vi "Data_Partitioning log.vi"() -> ()   [LabVIEW 2020]
uses:
  Global Variables/Trial_Flag.vi
  Global Variables/Global Send To ANN.vi
  Global Variables/Trainning Done.vi
  Global Variables/rating_done.vi
  Global Variables/Global User_Answer.vi
panel:
  out "Array of Single":sgl[][](array[numeric])
  out "Sended frame":dbl[](array[numeric])
  out "sorted 2D array":dbl[][](array[numeric])
  out "Open File":errorcluster
  out "Pre-Partition":dbl[][](array[numeric])
  in  "stop":bool
  # "Correct"
  # "Trial n"
  # "Window n"
  # "Timestamp"
  # "Left pupil"
  # "Right pupil"
  # "Label"
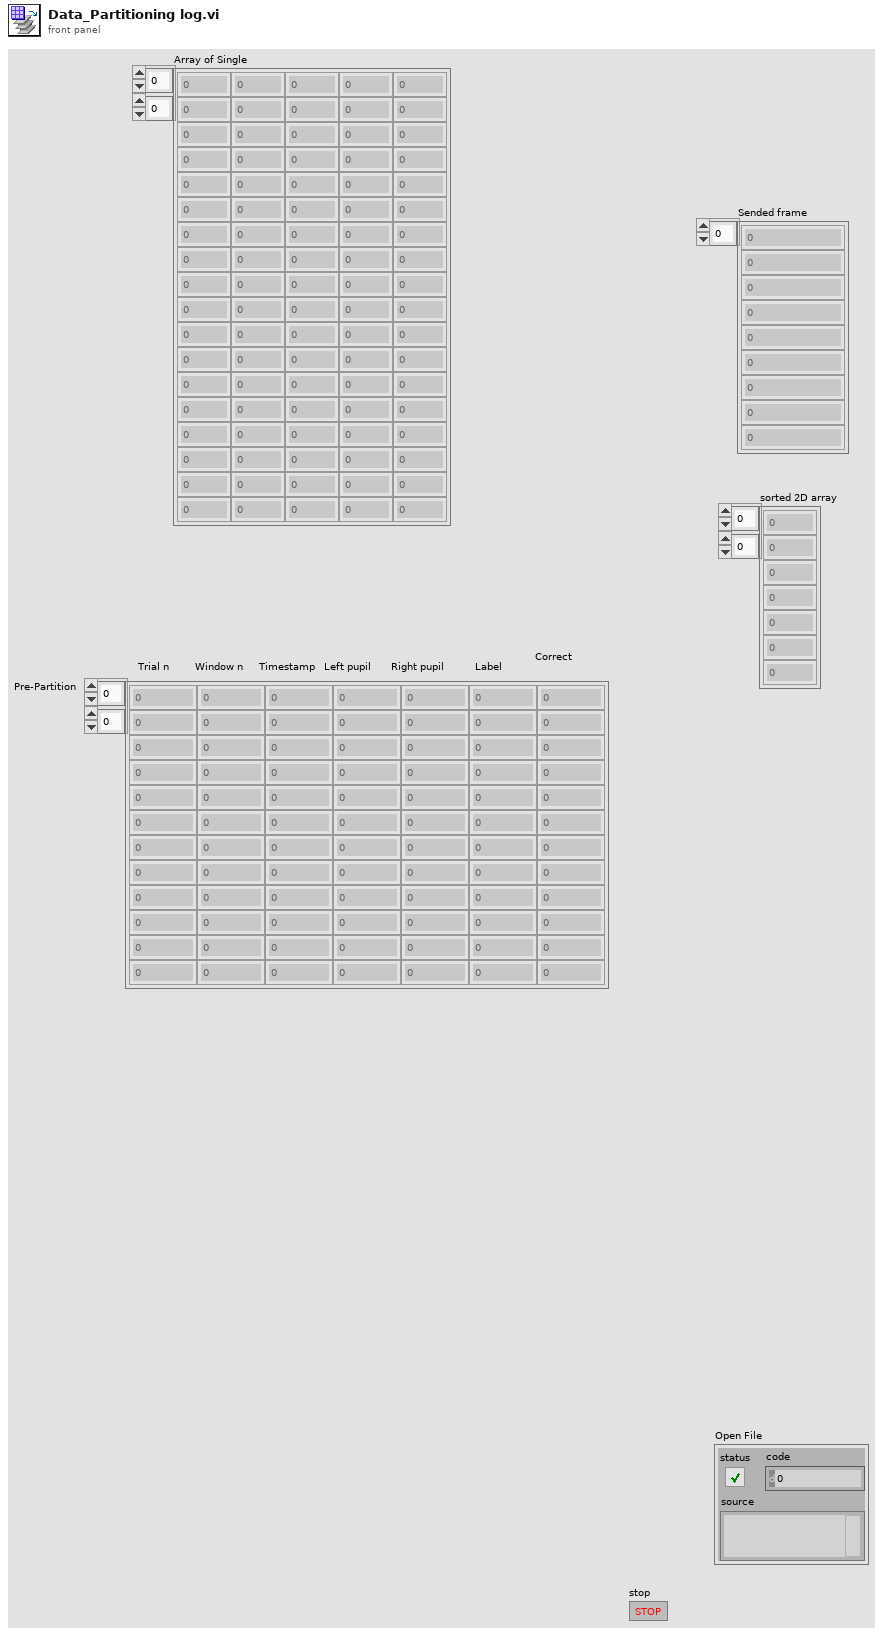
[diagram p1: front panel]
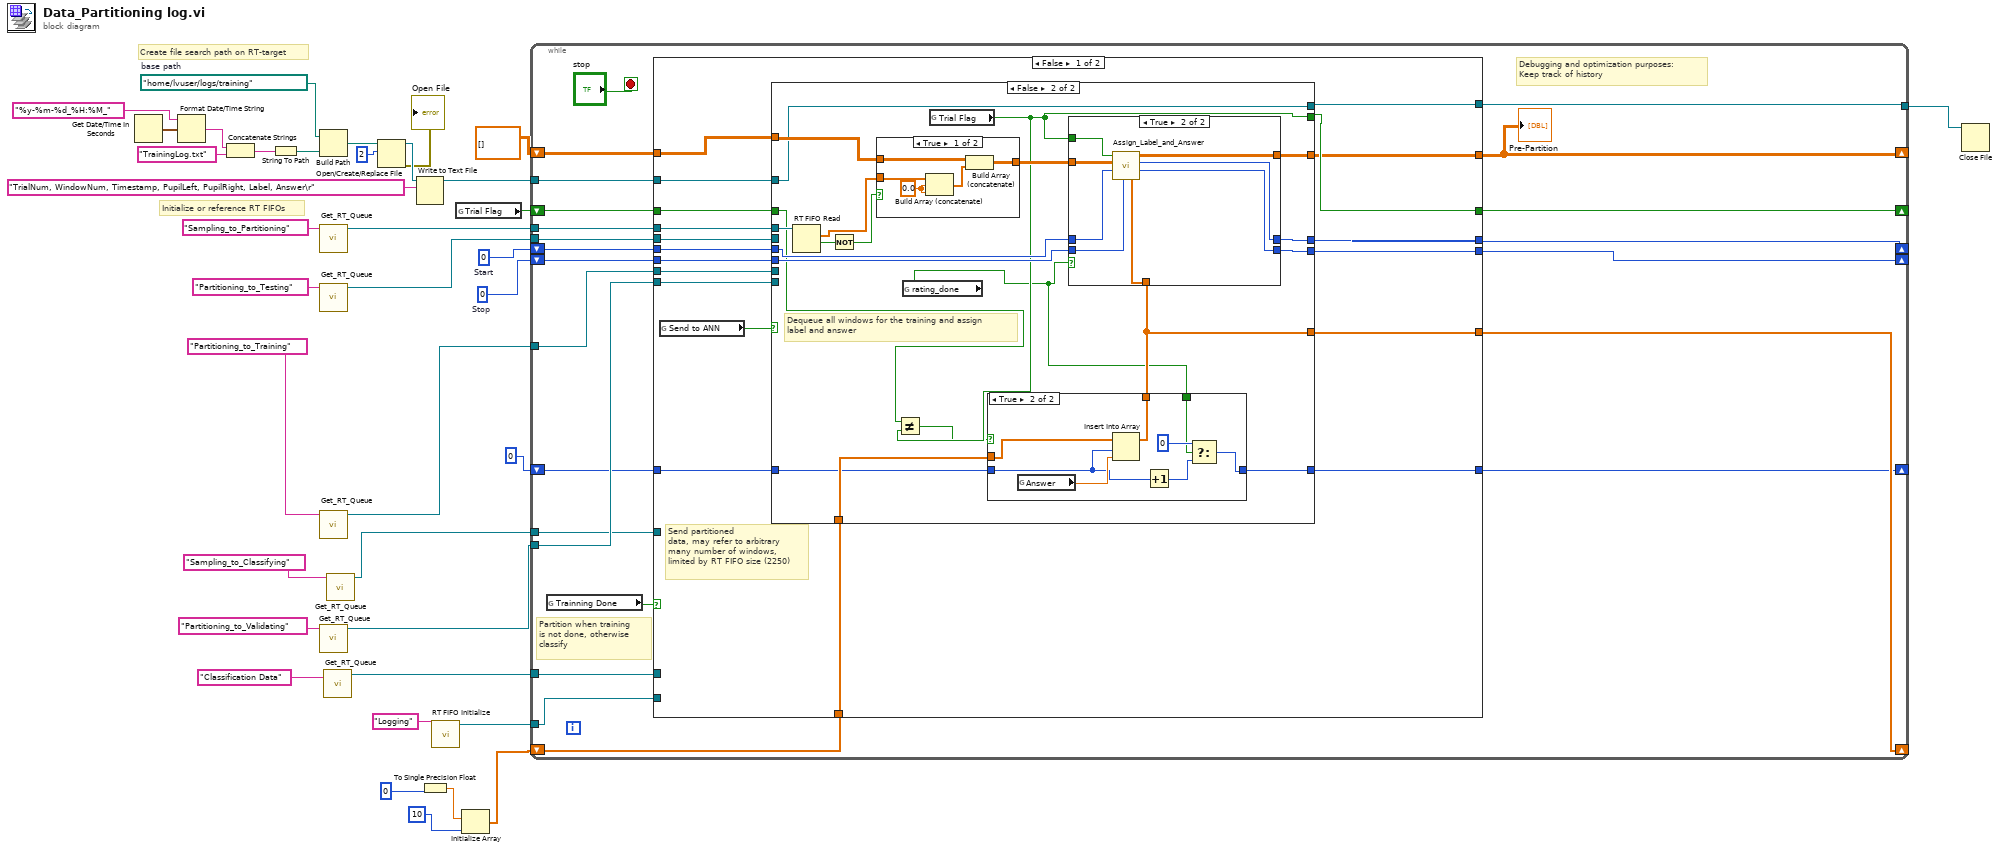
[diagram p0: block diagram]
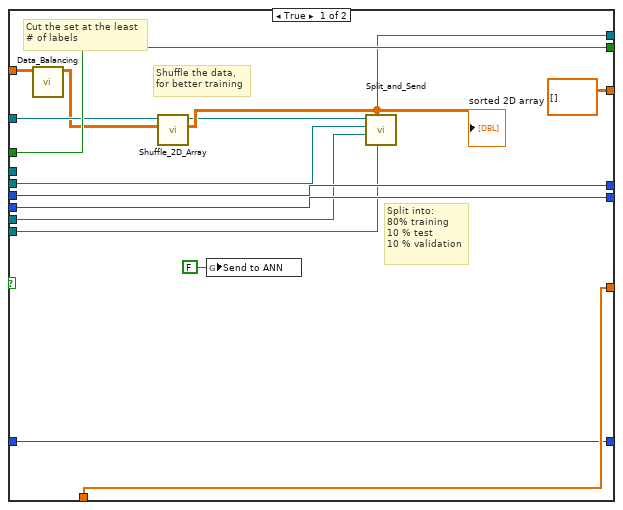
[diagram p2: hidden frame]
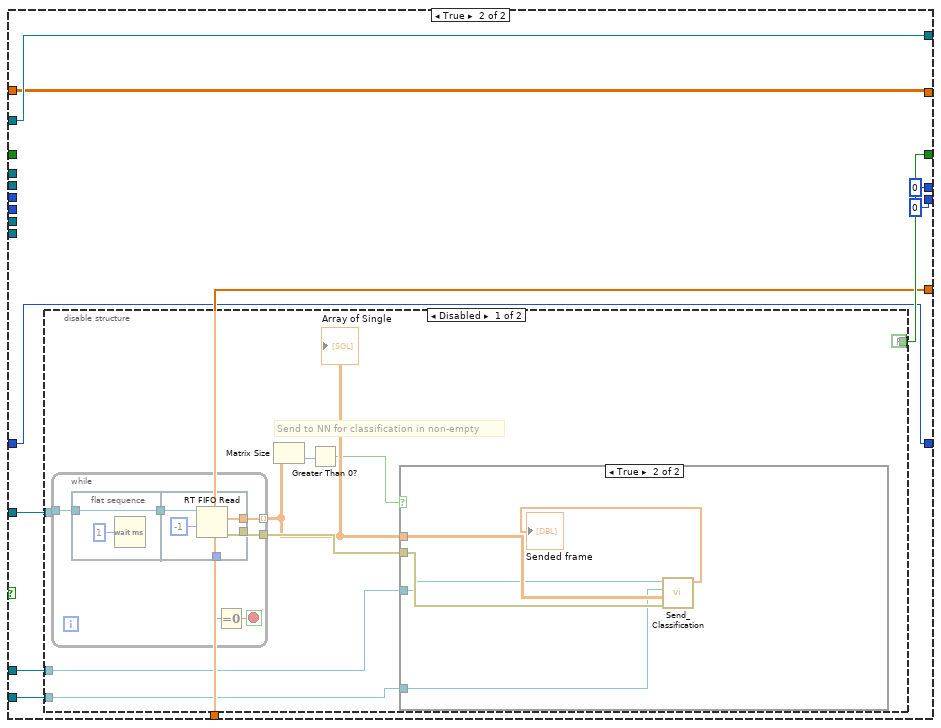
[diagram p6: hidden frame]
diagram:
  w32 = path "/home/lvuser/logs/training"  # base path
  w37 = 0  # Start
  w36 = 0  # Stop
  # "Initialize or reference RT FIFOs"
  # "Create file search path on RT-target"
  n1 = Get Date/Time In Seconds() -> (seconds since 1Jan1904=w25:timestamp)
  n2 = Format Date/Time String(time format string (%c)="%y-%m-%d_%H:%M_", seconds (now)=w25) -> (date/time string=w24:string)  [unwired: 1 in]
  n3 = Concatenate Strings(w24, "TrainingLog.txt") -> (w29:string)
  n4 = String To Path(string=w29) -> (path=w30:path)
  n5 = Build Path(base path=w32, name or relative path=w30) -> (appended path=w33:path)
  n6 = call "Get_RT_Queue.vi"("String"="Sampling_to_Partitioning") -> ("rt fifo single"=w13:refnum<k33>)  [unwired: 8 in, 2 out]
  n7 = call "Get_RT_Queue.vi"("String"="Partitioning_to_Testing") -> ("rt fifo single"=w15:refnum<k33>)  [unwired: 8 in, 2 out]
  n8 = call "Get_RT_Queue.vi"("String"="Partitioning_to_Training") -> ("rt fifo single"=w18:refnum<k33>)  [unwired: 8 in, 2 out]
  n9 = call "Get_RT_Queue.vi"("String"="Partitioning_to_Validating") -> ("rt fifo single"=w19:refnum<k33>)  [unwired: 8 in, 2 out]
  n10 = call "Get_RT_Queue.vi"("String"="Classification Data") -> ("rt fifo single"=w8:refnum<k33>)  [unwired: 8 in, 2 out]
  n11 = call "Get_RT_Queue.vi"("String"="Sampling_to_Classifying") -> ("rt fifo single"=w9:refnum<k33>)  [unwired: 8 in, 2 out]
  n12 = Open/Create/Replace File(file path (use dialog)=w33, operation (0:open)=2) -> (refnum out=w34:refnum<file>, error out=→"Open File":errorcluster)  [unwired: 4 in, 1 out]
  n13 = Write to Text File(file (use dialog)=w34, text="TrialNum, WindowNum, Timestamp, PupilLeft, PupilRight, Label, Answer\r") -> (refnum out=w27:refnum<file>)  [unwired: 2 in, 2 out]
  n14 = To Single Precision Float(number=0) -> (single precision float=w3:sgl)
  n15 = call "RT FIFO Initialize.vi"("name (unnamed)"="Logging") -> ("rt fifo"=w6:refnum<k33>)  [unwired: 9 in, 1 out]
  n16 = global read "Trial_Flag.vi" "Trial Flag"() -> (w35:bool)
  n17 = Initialize Array(w3, 10) -> (w2:sgl[])
  n18 = while {
    shift-right: [w47] -> _
    shift-left: sgl[][] [] -> [w60]
    shift-right: [w57] -> _
    shift-left: w37 -> [w55]
    shift-right: [w58] -> _
    shift-left: w36 -> [w46]
    shift-right: [w54] -> _
    shift-left: w35 -> [w56]
    tunnel: w13 -> [w53]
    tunnel: w18 -> [w52]
    tunnel: w15 -> [w51]
    tunnel: w19 -> [w50]
    tunnel: w27 -> [w49]
    tunnel: [w48] -> w22
    tunnel: w8 -> [w44]
    tunnel: w9 -> [w43]
    tunnel: w6 -> [w42]
    shift-right: [w39] -> _
    shift-left: w2 -> [w41]
    shift-right: [w38] -> _
    shift-left: 0 -> [w40]
    stop <- "stop" stop-if-true
    # "Debugging and optimization purposes: \nKeep track of history"
    # "Partition when training \nis not done, otherwise \nclassify"
    n19 = global read "Trainning Done.vi" "Trainning Done"() -> (w45:bool)
    n20 = case shown="False" w45 {
      tunnel: w60 -> [w79 w148]
      tunnel: [w78 0 ("Start out")] -> w58
      tunnel: [w77 0 ("Stop out")] -> w57
      tunnel: w56 -> [w76 _]
      tunnel: w55 -> [w75 _]
      tunnel: [w74 w150] -> w54
      tunnel: w53 -> [w73 _]
      tunnel: w52 -> [w72 _]
      tunnel: w51 -> [w71 _]
      tunnel: w50 -> [w70 _]
      tunnel: w49 -> [w69 w149]
      tunnel: [w68 w149] -> w48
      tunnel: [w67 w148] -> w47
      tunnel: w46 -> [w66 _]
      tunnel: w44 -> [_ w146]
      tunnel: w43 -> [_ w147]
      tunnel: w42 -> [_ w145]
      tunnel: w41 -> [w64 w144]
      tunnel: w40 -> [w63 w143]
      tunnel: [w62 w144] -> w39
      tunnel: [w61 w143] -> w38
      frame False {
        # "Send partitioned \ndata, may refer to arbitrary \nmany number of windows, \nlimited by RT FIFO size (2250)"
        n21 = global read "Global Send To ANN.vi" "Send to ANN"() -> (w65:bool)
        n22 = case shown="False" w65 {
          tunnel: w79 -> [w85 w115]
          tunnel: [w94 w113] -> w78
          tunnel: [sgl[][] [] ("Array out") w112] -> w67
          tunnel: [w93 w111] -> w77
          tunnel: w76 -> [w95 w103]
          tunnel: w75 -> [w93 w110]
          tunnel: w66 -> [w94 w109]
          tunnel: [w95 w102] -> w74
          tunnel: w73 -> [_ w108]
          tunnel: w72 -> [w92 _]
          tunnel: w71 -> [w91 _]
          tunnel: w70 -> [w90 _]
          tunnel: w69 -> [w88 w106]
          tunnel: [w86 w106] -> w68
          tunnel: w64 -> [w81 w100]
          tunnel: w63 -> [w80 w99]
          tunnel: [w81 w98] -> w62
          tunnel: [w80 w97] -> w61
          frame True {
            # "Split into: \n80% training \n10 % test \n10 % validation"
            # "Shuffle the data, \nfor better training"
            # "Cut the set at the least \n# of labels"
            n23 = call "Data_Balancing.vi"("Array in"=w85) -> ("Array out"=w84:sgl[][])  [unwired: 10 in]
            n24 = call "Shuffle_2D_Array.vi"("Array"=w84, "Byte Stream File in"=w88) -> ("sorted 2D array"=w89:dbl[][], "Byte Stream File out"=w87:refnum<file>)  [unwired: 8 in]
            "sorted 2D array" <- w89
            n25 = global write "Global Send To ANN.vi" "Send to ANN"(FALSE ("Send to ANN")) -> ()
            n26 = call "Split_and_Send.vi"("rt fifo"=w90, "sorted 2D array"=w89, "rt fifo 3"=w92, "rt fifo 2"=w91, "Byte Stream File in"=w87) -> ("Byte Stream File out"=w86:refnum<file>)  [unwired: 6 in]
          }
          frame False {
            # "Dequeue all windows for the training and assign \nlabel and answer"
            n27 = RT FIFO Read(0:w108) -> (9:w107:sgl[], 10:w105:bool)  [unwired: 3 in, 3 out]
            n28 = Not(x=w105) -> (.not. x?=w104:bool)
            n29 = case shown="True" w104 {
              tunnel: w115 -> [w140 w142]
              tunnel: [w141 w142] -> w114
              tunnel: w107 -> [w139 _]
              frame True {
                w138 = sgl 0.0
                n30 = Build Array (concatenate)(w139, w138, w138) -> (w137:sgl[])
                n31 = Build Array (concatenate)(w140, w137) -> (w141:sgl[][])
              }
              frame False {
              }
            }
            n32 = global read "rating_done.vi" "rating_done"() -> (w96:bool)
            n33 = global read "Trial_Flag.vi" "Trial Flag"() -> (w102:bool)
            n34 = Not Equal?(x=w103, y=w102) -> (x != y?=w101:bool)
            n35 = case shown="True" w101 {
              tunnel: w100 -> [w116 w125]
              tunnel: w99 -> [w117 w121]
              tunnel: [w116 w123] -> w98
              tunnel: [w117 w119] -> w97
              tunnel: w96 -> [_ w118]
              frame False {
              }
              frame True {
                n36 = global read "Global User_Answer.vi" "Answer"() -> (w124:dbl)
                n37 = Insert Into Array(array=w125, index=w121, new element=w124) -> (w123:sgl[])
                n38 = Increment(x=w121) -> (x+1=w120:i32)
                n39 = Select(t=0, s=w118, f=w120) -> (s? t:f=w119:i32)
              }
            }
            n40 = case shown="True" w96 {
              tunnel: w114 -> [w128 w136]
              tunnel: w110 -> [w127 w132]
              tunnel: w109 -> [w126 w134]
              tunnel: [w126 w133] -> w113
              tunnel: [w128 w135] -> w112
              tunnel: [w127 w131] -> w111
              tunnel: w102 -> [_ w130]
              tunnel: w98 -> [_ w129]
              frame False {
              }
              frame True {
                n41 = call "Assign_Label_and_Answer.vi"("Start in"=w134, 8:w129, "Stop in"=w132, "Array in"=w136, "Trial Flag"=w130) -> ("Start out"=w133:i32, "Stop out"=w131:i32, "Array out"=w135:sgl[][])  [unwired: 4 in]
              }
            }
          }
        }
      }
      frame True {
        n42 = disable-structure shown="Disabled" {
          disable-tunnel: [FALSE ("Trial Flag") _] -> w150
          disable-tunnel: w147 -> [w155 _]
          disable-tunnel: w146 -> [w154 _]
          disable-tunnel: w145 -> [w153 _]
          frame Disabled {
            # "Send to NN for classification in non-empty"
            n43 = while {
              tunnel: w155 -> [w171]
              tunnel: [w169] -> w158 mode=indexing
              tunnel: [w168] -> w159
              stop <- w167 stop-if-true
              n44 = flat-sequence {
                tunnel: w171 -> [w173]
                tunnel: [w173] -> w166
                tunnel: [w177] -> w170
                tunnel: [w176] -> w169
                tunnel: [w175] -> w168
                tunnel: w166 -> [w178]
                frame #0 {
                  n45 = Wait (ms)(milliseconds to wait=u32 1) -> ()  [unwired: 1 out]
                }
                frame #1 {
                  n46 = RT FIFO Read(0:w178, 2:-1 ("timeout in ms (0)")) -> (7:w177:u32, 9:w176:sgl[], 11:w175:errorcluster)  [unwired: 2 in, 2 out]
                }
              }
              n47 = Equal To 0?(x=w170) -> (x = 0?=w167:bool)
            }
            "Array of Single" <- w158
            n48 = Matrix Size(0:w158) -> (2:w156:i32)  [unwired: 1 out]
            n49 = Greater Than 0?(x=w156) -> (x > 0?=w157:bool)
            n50 = case shown="True" w157 {
              tunnel: w158 -> [_ w165]
              tunnel: w159 -> [_ w164]
              tunnel: w154 -> [_ w163]
              tunnel: w153 -> [_ w162]
              frame False {
              }
              frame True {
                n51 = call "Send_Classification.vi"("error in (no error)"=w164, "Window"=w165, "logging FIFO"=w162, "Classification FIFO"=w163) -> ("Sended frame"=→"Sended frame":dbl[])  [unwired: 7 in]
              }
            }
          }
          frame Enabled {
          }
        }
      }
    }
    "Pre-Partition" <- w47
  }
  n52 = Close File(refnum=w22) -> ()  [unwired: 1 in, 2 out]
